vi "dfd_Get Initial Coefficients.vi"(7 "M":i32=4, 8 "error in (no error)":errorcluster, 10 "roll off":dbl=0.2, 11 "order":i32=-1) -> (0 "error out":errorcluster, 2 "dup roll off":dbl, 3 "initial h":dbl[](array[numeric]))   [LabVIEW 2017, in "NI_DigFilter_FilterBank.lvlib"]
uses:
  <vilib>/addons/Digital Filter Design/NI_DigFilter_FilterBank.lvlib
  <vilib>/addons/Digital Filter Design/_REMEZ.llb/remez_fir order and types.ctl
  <vilib>/addons/Digital Filter Design/_REMEZ.llb/remez_fir filter type.ctl
  <vilib>/addons/Digital Filter Design/_REMEZ.llb/remez_single band description.ctl
  <vilib>/addons/Digital Filter Design/NI_DigFilter_Design.lvlib
  <vilib>/addons/Digital Filter Design/NI_DigFilterLicensed.lvlib
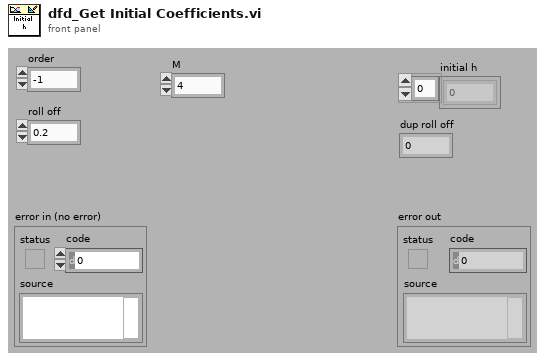
[diagram p1: front panel]
types:
  T1 = typedef "remez_fir order and types.ctl" = cluster{"# of taps":i32, "filter type":T2, "minimum order":enum32{"user defined", "minEven", "minOdd"}}
  T2 = typedef "NI_DigFilterLicensed.lvlib/remez_fir filter type.ctl" = enum32{"Symmetric", "Antisymmetric", "Differentiator", "Hilbert", "Minimum Phase", "Maximum Phase"}
  T3 = typedef "remez_single band description.ctl" = cluster{"points":cluster{"f":dbl, "A":dbl, "W":dbl, "forced gain?":bool}[], "band weight":dbl, "constraint":dbl, "ripple idx":i32, "in band weight option":enum16{"ignore", "linear interpolation", "const amplitude %"}}
  T4 = cluster{"fpass":dbl, dbl, dbl, "forced gain?":bool}
  T5 = cluster{"fstop":dbl, dbl, dbl, "forced gain?":bool}
  T6 = cluster{"fpass":dbl, dbl, dbl, "forced gain?":bool}[]
  T7 = cluster{"fstop":dbl, dbl, dbl, "forced gain?":bool}[]
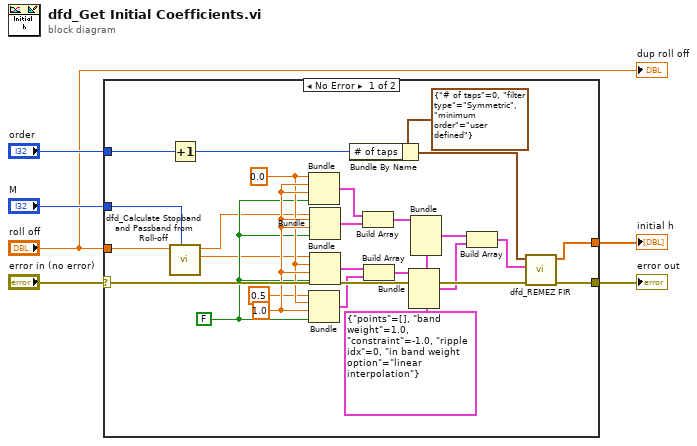
[diagram p0: block diagram]
diagram:
  n1 = case shown="No Error" "error in (no error)" {
    selector: "error in (no error)" -> [w30 w32]
    tunnel: "roll off" -> [w9 _]
    tunnel: "M" -> [w10 _]
    tunnel: [w28 _] -> w1
    tunnel: "order" -> [w31 _]
    tunnel: [w29 w32] -> w4
    frame No Error {
      w12 = T3 {"points"=[], "band weight"=1.0, "constraint"=-1.0, "ripple idx"=0, "in band weight option"=enum."linear interpolation"} ("band")
      w13 = FALSE ("forced gain?")
      w27 = 1.0
      w21 = 0.0
      n2 = Increment(x=w31) -> (x+1=w14:i32)
      n3 = call <vilib>:"dfd_Calculate Stopband and Passband from Roll-off.vi"("#channel"=w10, "roll off"=w9) -> ("fstop"=w7:dbl, "fpass"=w8:dbl)  [unwired: 8 in]
      n4 = Bundle(w21, w27, w27, "forced gain?"=w13) -> (w17:cluster{dbl, dbl, dbl, "forced gain?":bool})  [unwired: 1 in]
      n5 = Bundle(0.5, w21, w27, "forced gain?"=w13) -> (w23:cluster{dbl, dbl, dbl, "forced gain?":bool})  [unwired: 1 in]
      n6 = Bundle("fpass"=w8, w27, w27, "forced gain?"=w13) -> (w18:T4)  [unwired: 1 in]
      n7 = Bundle("fstop"=w7, w21, w27, "forced gain?"=w13) -> (w24:T5)  [unwired: 1 in]
      n8 = Bundle By Name(cluster=T1 {"# of taps"=0, "filter type"=enum."Symmetric", "minimum order"=enum."user defined"} ("order and type"), "# of taps"=w14) -> (w16:T1)
      n9 = Build Array(w17, w18) -> (w19:T6)
      n10 = Build Array(w24, w23) -> (w22:T7)
      n11 = Bundle(cluster=w12, "points"=w22) -> (w26:T3)  [unwired: 4 in]
      n12 = Bundle(cluster=w12, "points"=w19) -> (w25:T3)  [unwired: 4 in]
      n13 = Build Array(w25, w26) -> (w11:T3[])
      n14 = call <vilib>:"dfd_REMEZ FIR.vi"("error in (no error)"=w30, "band specification"=w11, "order and type"=w16) -> ("error out"=w29:errorcluster, "h"=w28:dbl[])  [unwired: 5 in, 2 out]
    }
    frame Error {
    }
  }
  "initial h" <- w1
  "error out" <- w4
  "dup roll off" <- "roll off"
